vi "get_info.vi"(8 "error in (no error)":errorcluster, 11 "TCP Connection in":refnum<class "TCP Connection.lvclass">) -> (0 "error out":errorcluster, 2 "info.":string, 3 "TCP Connection out":refnum<class "TCP Connection.lvclass">)   [LabVIEW 2019, in "TCP Connection.lvclass"]
uses:
  TCP Connection.lvclass
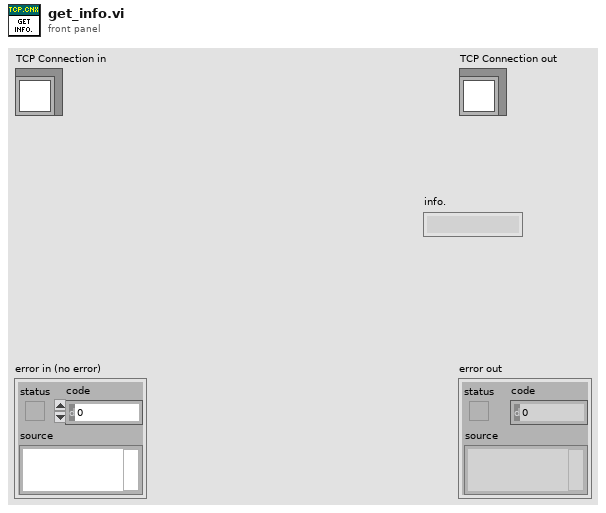
[diagram p1: front panel]
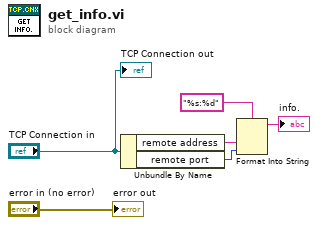
[diagram p0: block diagram]
diagram:
  n1 = Unbundle By Name("TCP Connection in") -> ("remote address"=w3:string, "remote port"=w2:u16)
  n2 = Format Into String(format string="%s:%d", w3, w2) -> (resulting string=→"info.":string)  [unwired: 2 in, 1 out]
  "error out" <- "error in (no error)"
  "TCP Connection out" <- "TCP Connection in"
